vi "VITree.vi"   [LabVIEW 2016, in "Drona Test.lvlib"]
uses:
  Drona Test.lvlib
  main/apis/Assert/AssertControlValue/AlmostEqual.vi
  main/apis/Assert/AssertControlValue/Equal.vi
  main/apis/Assert/AssertControlValue/NotEqual.vi
  main/apis/Assert/AssertControlValue/Greater.vi
  main/apis/Assert/AssertControlValue/GreaterOrEqual.vi
  main/apis/Assert/AssertControlValue/Less.vi
  main/apis/Assert/AssertControlValue/LessOrEqual.vi
  main/apis/Assert/AssertControlValue/True.vi
  main/apis/Assert/AssertControlValue/False.vi
  main/apis/Assert/AssertControlDisable/AssertDisabled.vi
  main/apis/Assert/AssertControlDisable/AssertDisabledAndGrayedOut.vi
  main/apis/Assert/AssertControlDisable/AssertEnabled.vi
  main/apis/Setup/GetControlValue/GetControlValueByPathString.vi
  main/apis/Setup/GetControlRef/GetControlRefByArray.vi
  main/apis/Setup/GetVI/GetVIByName.vi
  main/apis/Setup/GetVI/GetVIByPath.vi
  main/apis/Stimulus/ValueSignal/ValueSignalByPathString.vi
  main/apis/Stimulus/ValueSignal/ValueSignalByPathArray.vi
  main/Drona.lvlib
  main/apis/Setup/GetVI/GetVI.lvlib
  main/apis/Setup/GetControlValue/GetControlValue.lvlib
  main/apis/Setup/GetControlRef/GetControlRef.lvlib
  main/apis/Stimulus/VI/VI.lvlib
  main/apis/Stimulus/ValueSignal/ValueSignal.lvlib
  main/apis/Assert/AssertControlValue/AssertControlValue.lvlib
  main/apis/Assert/AssertControlDisable/AssertControlDisable.lvlib
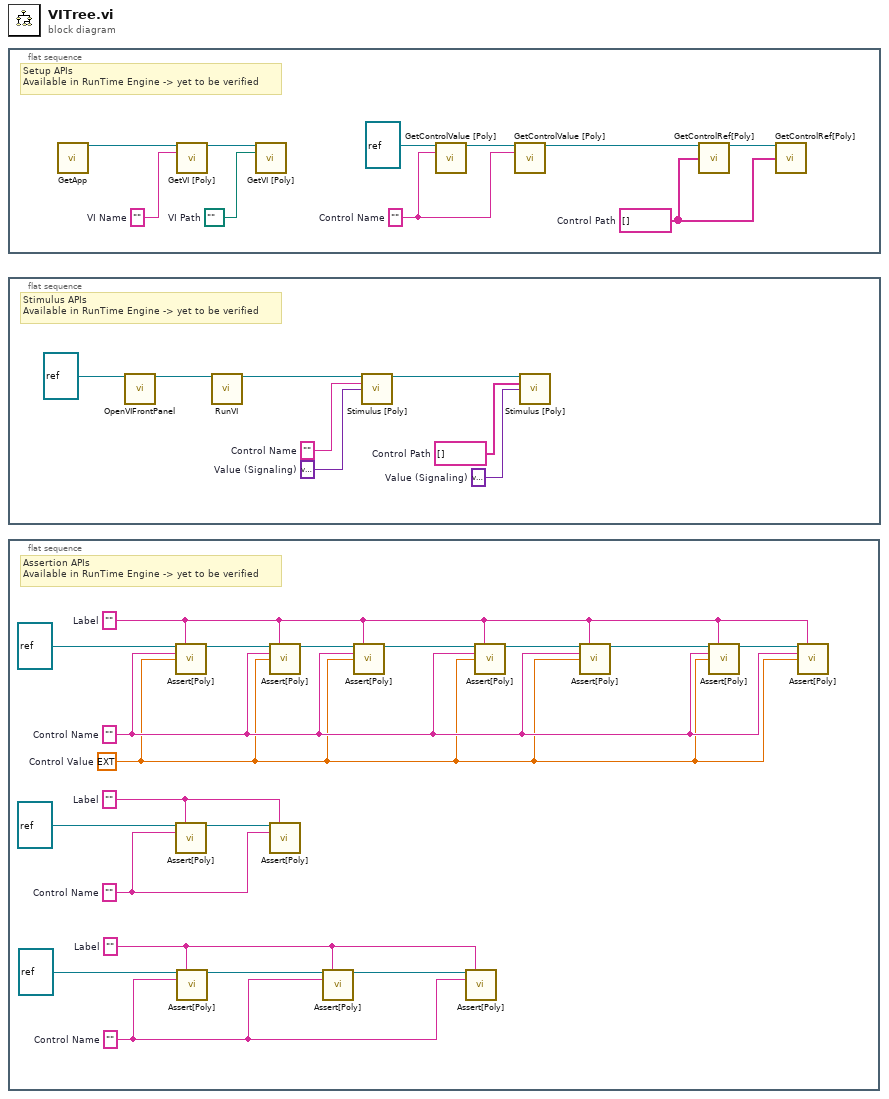
[diagram p0: block diagram]
diagram:
  n1 = flat-sequence {
    frame #0 {
      w1 = string[] []  # Control Path
      w2 = ""  # Control Name
      w7 = path ""  # VI Path
      w8 = ""  # VI Name
      # "Setup APIs\nAvailable in RunTime Engine -> yet to be verified"
      n2 = call "GetApp.vi"() -> ("Application Ref"=w9:refnum<vi>)  [unwired: 14 in, 1 out]
      n3 = call-poly "GetVI [Poly].vi"("Application Ref in"=w9, "VI Name"=w8) -> ("Application Ref out"=w10:refnum<vi>)  [unwired: 11 in, 2 out]
      n4 = call-poly "GetVI [Poly].vi"("Application Ref in"=w10, "VI Path"=w7) -> ()  [unwired: 11 in, 3 out]
      n5 = call-poly "GetControlValue [Poly].vi"("VI Reference In"=refnum<vi> refnum, "Control Path"=w2) -> ("VI Reference Out"=w4:refnum<vi>)  [unwired: 11 in, 2 out]
      n6 = call-poly "GetControlValue [Poly].vi"("VI Reference In"=w4, "Control Path"=w2) -> ("VI Reference Out"=w5:refnum<vi>)  [unwired: 11 in, 2 out]
      n7 = call-poly "GetControlRef[Poly].vi"("VI Reference In"=w5, "Control Path"=w1) -> ("VI Reference Out"=w6:refnum<vi>)  [unwired: 11 in, 2 out]
      n8 = call-poly "GetControlRef[Poly].vi"("VI Reference In"=w6, "Control Path"=w1) -> ()  [unwired: 11 in, 3 out]
    }
  }
  n9 = flat-sequence {
    frame #0 {
      w11 = variant  # Value (Signaling)
      w12 = string[] []  # Control Path
      w14 = variant  # Value (Signaling)
      w15 = ""  # Control Name
      # "Stimulus APIs\nAvailable in RunTime Engine -> yet to be verified"
      n10 = call "OpenVIFrontPanel.vi"("VI Reference In"=refnum<vi> refnum) -> ("VI Reference Out"=w17:refnum<vi>)  [unwired: 13 in, 1 out]
      n11 = call "RunVI.vi"("VI Reference In"=w17) -> ("VI Reference Out"=w16:refnum<vi>)  [unwired: 13 in, 1 out]
      n12 = call-poly "Stimulus [Poly].vi"("VI Reference In"=w16, "Control Path"=w15, "Value (Signaling)"=w14) -> ("VI Reference Out"=w13:refnum<vi>)  [unwired: 11 in, 1 out]
      n13 = call-poly "Stimulus [Poly].vi"("VI Reference In"=w13, "Control Path"=w12, "Value (Signaling)"=w11) -> ()  [unwired: 11 in, 2 out]
    }
  }
  n14 = flat-sequence {
    frame #0 {
      w19 = ""  # Control Name
      w20 = ""  # Label
      w27 = ""  # Control Name
      w26 = ""  # Label
      w28 = ext 0.0  # Control Value
      w29 = ""  # Control Name
      w30 = ""  # Label
      # "Assertion APIs\nAvailable in RunTime Engine -> yet to be verified"
      n15 = call-poly "Assert[Poly].vi"("VI Reference In"=refnum<vi> refnum, "Label"=w30, "Control Path"=w29, "Control Value"=w28) -> ("VI Reference Out"=w36:refnum<vi>)  [unwired: 10 in, 1 out]
      n16 = call-poly "Assert[Poly].vi"("VI Reference In"=refnum<vi> refnum, "Label"=w26, "Control Path"=w27) -> ("VI Reference Out"=w25:refnum<vi>)  [unwired: 11 in, 1 out]
      n17 = call-poly "Assert[Poly].vi"("VI Reference In"=refnum<vi> refnum, "Label"=w20, "Control Path"=w19) -> ("VI Reference Out"=w22:refnum<vi>)  [unwired: 11 in, 1 out]
      n18 = call-poly "Assert[Poly].vi"("VI Reference In"=w36, "Label"=w30, "Control Path"=w29, "Control Value"=w28) -> ("VI Reference Out"=w35:refnum<vi>)  [unwired: 10 in, 1 out]
      n19 = call-poly "Assert[Poly].vi"("VI Reference In"=w25, "Label"=w26, "Control Path"=w27) -> ()  [unwired: 11 in, 2 out]
      n20 = call-poly "Assert[Poly].vi"("VI Reference In"=w22, "Label"=w20, "Control Path"=w19) -> ("VI Reference Out"=w21:refnum<vi>)  [unwired: 11 in, 1 out]
      n21 = call-poly "Assert[Poly].vi"("VI Reference In"=w35, "Label"=w30, "Control Path"=w29, "Control Value"=w28) -> ("VI Reference Out"=w34:refnum<vi>)  [unwired: 10 in, 1 out]
      n22 = call-poly "Assert[Poly].vi"("VI Reference In"=w21, "Label"=w20, "Control Path"=w19) -> ()  [unwired: 11 in, 2 out]
      n23 = call-poly "Assert[Poly].vi"("VI Reference In"=w34, "Label"=w30, "Control Path"=w29, "Control Value"=w28) -> ("VI Reference Out"=w33:refnum<vi>)  [unwired: 10 in, 1 out]
      n24 = call-poly "Assert[Poly].vi"("VI Reference In"=w33, "Label"=w30, "Control Path"=w29, "Control Value"=w28) -> ("VI Reference Out"=w32:refnum<vi>)  [unwired: 10 in, 1 out]
      n25 = call-poly "Assert[Poly].vi"("VI Reference In"=w32, "Label"=w30, "Control Path"=w29, "Control Value"=w28) -> ("VI Reference Out"=w31:refnum<vi>)  [unwired: 10 in, 1 out]
      n26 = call-poly "Assert[Poly].vi"("VI Reference In"=w31, "Label"=w30, "Control Path"=w29, "Control Value"=w28) -> ()  [unwired: 10 in, 2 out]
    }
  }
